vi "CALC_CUST_MOD.vi"(0 "VISA IN":refnum<visa-resource-name>, 1 "Parameter to change Measurement":string, 5 "error in":errorcluster, 7 "Channel":i32) -> (14 "VISA Out":refnum<visa-resource-name>, 19 "error out":errorcluster)   [LabVIEW 2018, in "PNA-X.lvlib"]
doc: "CALCulate<cnum>:CUSTom:MODify <param> \n1493\n\n(Write-only) Changes the selected custom measurement to a different parameter. \nSee an example using this command for a VMC and SMC measurement \nParameters \n<cnum> Channel of the custom measurement to be changed. First, select the \nmeasurement using CALC:PAR:SEL. \n<param> Parameter to change the custom measurement to. Select a parameter that is \nvalid for the type of measurement. \nType Valid Parameters \nVMC Measurement \"S11\" \n\"VC21\" \n\"S22\" \nSMC Measurement \"S11\" \n\"SC21\" \n\"SC12\" \n\"S22\" \n\"Ipwr\" \n\"RevIPwr\" \n\"Opwr\" \n\"RevOPwr\" \nExamples SYST:PRES \nCALC2:CUST:DEF 'My VC21', 'Vector Mixer/Converter' \nCALC:PAR:SEL 'My VC21' \nCALC2:CUST:MOD 'S22' \nQuery Syntax Not applicable \nOverlapped? No \nDefault Not applicable \n1494\n\n1495\n\nCalculate:Data Commands \nControls writing and reading PNA measurement data. \nClick on a blue keyword to view the command details. \nSee Also \nExample Programs \nData Access Map \nSynchronizing the PNA and Controller \nTo read receiver data, use CALC:RDATA? \nTo read error terms, use SENS:CORR:CSET:DATA \nTo read SnP measurement data, use CALC:DATA:SNP? \nSCPI Command Tree \nCritical Note: CALCulate commands act on the selected measurement. You can select one \nmeasurement for each channel using Calc:Par:Select \n(Write) CALCulate<cnum>:DATA <char>,<data> \n(Read) CALCulate<cnum>:DATA? <char> \nReads or writes Measurement data, Memory data, or Normalization Divisor data from the Data \nAccess Map location. \nFor Measurement data, use FDATA or SDATA \nFor Memory data, use FMEM or SMEM. When querying memory, you must first store a trace into memory \nusing CALC:MATH:MEMorize. \nFor Normalization Divisor (Receiver Power Cal error term) data, use SDIV \n1496\n\nFor write operations, data type depends on FORM:DATA command. \nNote: The Calc:Data SCORR command to read / write error terms is Superseded with \nSENS:CORR:CSET:DATA. SCORR commands do NOT accommodate greater than 12 error terms. \nSee Critical Note \nParameters \n<cnum> Channel number of the measurement. There must be a selected measurement on that \nchannel. If unspecified, <cnum> is set to 1. \n<char> FDATA Formatted measurement data to or from Data Access Map location \nDisplay (access point 2). \nCorrected data is returned when correction is ON. \nUncorrected data is returned when correction is OFF. \nReturns TWO numbers per data point for Polar and Smith Chart format. \nReturns one number per data point for all other formats. \nFormat of the read data is same as the displayed format. \nSDATA Complex measurement data. \nWrites data to Data Access Map location Raw Measurement (access \npoint 0). \nWhen writing corrected data, and correction is ON, it will be corrected \nagain, resulting in meaningless data. \nReads data from Apply Error Terms (access point 1). \nReturns TWO numbers per data point. \nCorrected data is returned when correction is ON. \nUncorrected data is returned when correction is OFF. \nFMEM Formatted memory data to or from Data Access Map location Memory \nresult (access point 4). \nReturns TWO numbers per data point for Polar and Smith Chart format. \nReturns one number per data point for all other formats. \nFormat of the read data is same as the displayed format. \nReturned data reflects the correction level (On|OFF) when the data was \n1497\n\nstored into memory. \nSMEM Complex measurement data to or from Data Access Map location \nMemory (access point 3). \nReturns TWO numbers per data point. \nReturned data reflects the correction level (On|OFF) when the data was \nstored into memory. \nReturned data reflects the correction level (On|OFF) when the data was \nstored into memory. \nSDIV Complex data from Data Access Map location Normalization (5). \nReturns TWO numbers per data point. \nIf normalization interpolation is ON and the number of points changes \nafter the initial normalization, the divisor data will then be interpolated. \nWhen querying the normalization divisor, you must first store a divisor \ntrace using CALC:NORMalize[:IMMediate]. \nThe following Calc:Data SCORR command to read / write error terms is Superseded with \nSENS:CORR:CSET:DATA. These SCORR commands do NOT accommodate greater than 12 error \nterms. \nFor 2-Port \nSOLT and \nTRL \ncalibrations \nSpecify this \n<char> \nto get or put this Error Term... \nSCORR1 Forward Directivity \nSCORR2 Forward Source Match \nSCORR3 Forward Reflection Tracking \nSCORR4 Forward Isolation \nSCORR5 Forward Load Match \nSCORR6 Forward Transmission Tracking \nSCORR7 Reverse Directivity \nSCORR8 Reverse Source Match \nSCORR9 Reverse Reflection Tracking \nSCORR10 Reverse Isolation \nSCORR11 Reverse Load Match \nSCORR12 Reverse Transmission Tracking \n1498\n\nEXAMPLE \nCALC:DATA FDATA,Data(x) \ncalculate2:data sdata,data(r,i) \nSee another example using this command. \nReturn Type: Block data \nDefault - Not Applicable"
uses:
  PNA-X.lvlib
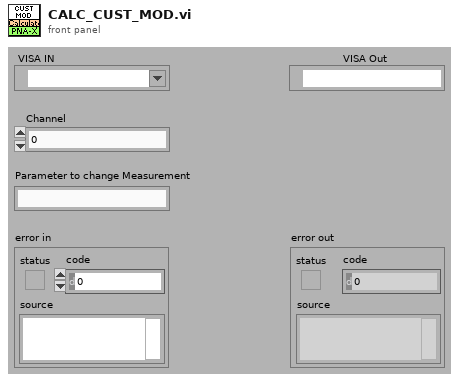
[diagram p1: front panel]
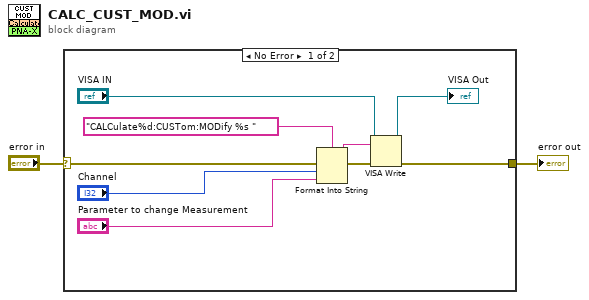
[diagram p0: block diagram]
diagram:
  n1 = case shown="No Error" "error in" {
    selector: "error in" -> [w11 w12]
    tunnel: [w6 w12] -> w1
    frame No Error {
      n2 = Format Into String(format string="CALCulate%d:CUSTom:MODify %s " ("Cmdline"), error in=w11, "Channel", "Parameter to change Measurement") -> (resulting string=w9:string, error out=w10:errorcluster)  [unwired: 1 in]
      n3 = VISA Write(VISA resource name="VISA IN", write buffer=w9, error in (no error)=w10) -> (VISA resource name out=→"VISA Out":refnum<visa-resource-name>, error out=w6:errorcluster)  [unwired: 1 out]
    }
    frame Error {
    }
  }
  "error out" <- w1
